vi "Module Execution Main.vi"(8 "error in":errorcluster, 10 "response queue":T1, 11 "command queue":T1) -> (0 "error out":errorcluster)   [LabVIEW 2013, in "module execution process.lvlib"]
doc: "This process allows a user to initialize, start, stop, monitor, and repeat using a message queue without stopping the main application. This process can be useful when you want to support the control of this target by one or more connected hosts."
uses:
  module execution process.lvlib
  <vilib>/NI/AMC/Message Queue.ctl
  <vilib>/NI/AMC/Message.ctl
  <vilib>/NI/Tools/Keyed Array/KeyedArray.ctl
  <vilib>/NI/Module Execution Interface/Engine Runtime/Engine Runtime Interface.lvclass
  <vilib>/NI/Configuration Framework/class discovery singleton/class discovery singleton methods.ctl
  SubVIs/configuration elements.ctl
  <vilib>/NI/Tag Bus Data Framework/Framework Configuration Classes/platypus configuration/engines cluster.ctl
  <vilib>/NI/Module Execution Interface/Engine Configuration/engine configuration.lvclass
  <vilib>/NI/Tag Bus Module Framework/module configuration/TBM module configuration.lvclass
  <vilib>/NI/Tag Bus Module Framework/runtime/TBM module execution interface.lvclass
  SubVIs/engine status data.ctl
  <vilib>/NI/Module Execution Interface/Engine Runtime/Execution States.ctl
  <vilib>/NI/AMC/Read Termination Message.vi
  <vilib>/NI/AMC/Create Single Message.vi
  <vilib>/NI/AMC/Globals.vi
  <vilib>/NI/Configuration Framework/class discovery singleton/class discovery singleton.lvlib
  <vilib>/NI/AMC/AMC.lvlib
  <vilib>/NI/Tag Bus Module Framework/FPGA manager/methods.ctl
  <vilib>/NI/Tag Bus Module Framework/FPGA manager/FPGA manager.lvlib
  <vilib>/userdefined/High Color/nirio_resource_hc.ctl
  <vilib>/rvi/interface/nirviOpenFPGA/nirviOpenFPGA.xnode
  <vilib>/NI/Tag Bus Data Framework/Framework Configuration Classes/target runtime/PL_Target Runtime.lvclass
  <vilib>/NI/Tag Bus Data Framework/Framework Configuration Classes/platypus configuration/PLConfigurationSerializer.lvlib
  <vilib>/NI/Configuration Framework/tree serializer/NISE_CEF_TreeSerializer.lvlib
  <vilib>/NI/Tag Bus Data Framework/Framework Configuration Classes/flattened data interface/PL_Serialization Interface.lvlib
  <vilib>/NI/Tools/Keyed Array/Tools_KeyedArray.lvlib
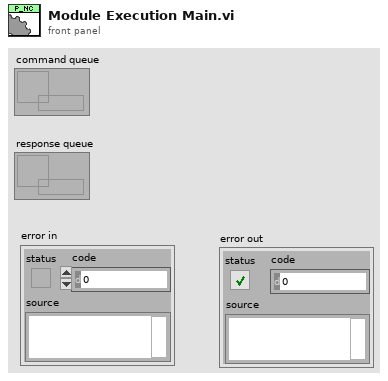
[diagram p1: front panel]
types:
  T1 = typedef "AMC.lvlib/Message Queue.ctl" = refnum<queue>
  T2 = typedef "class discovery singleton.lvlib/class discovery singleton methods.ctl" = enum16{"add search paths", "load class by name", "list available classes", "get class path"}
  T3 = typedef "module execution process.lvlib/configuration elements.ctl" = cluster{"Name":string, "opened?":bool, "configuration":T4, "engine":refnum<class "Engine Runtime Interface.lvclass">, "modules":refnum<class "TBM module execution interface.lvclass">[]}
  T4 = typedef "PLConfigurationSerializer.lvlib/engines cluster.ctl" = cluster{"engine configuration":refnum<class "engine configuration.lvclass">, "modules":refnum<class "TBM module configuration.lvclass">[]}
  T5 = typedef "nirio_resource_hc.ctl" = tag
  T6 = typedef "FPGA manager.lvlib/methods.ctl" = enum16{"initialize bitfile", "cache bitfile", "locate bitfile", "close bitfile"}
  T7 = typedef "module execution process.lvlib/engine status data.ctl" = cluster{"Name":string, "Engine State":T8, "Engine Error":errorcluster}
  T8 = typedef "Engine Runtime Interface.lvclass/Execution States.ctl" = enum16{"Initializing", "Paused (Initialized)", "Running", "Set Safe Outputs", "Uninitializing", "Stopped (Uninitialized)", "Error (Uninitialized)", "Safe State (Uninitialized)", "Closed"}
  T9 = typedef "module execution process.lvlib/command commands to rtexe process.ctl" = enum16{"Initialize", "Load from File", "Load from String", "Open All Engines", "Open Single Engine", "Initialize All Engines", "Initialize Single Engine", "Start All", "Start Single", "Pause All", "Pause Single", "Stop All", "Stop Single", "Close All", "Close Single", "Set Safe State All", "Set Safe State Single", "Get Status", "Exit", "Error", "Load Bitfile", "Unload Bitfile", "Add Search Paths"}
  T10 = typedef "NISE_CEF_TreeSerializer.lvlib/base file format.ctl" = cluster{"version":string, "data":string}
  T11 = typedef "NISE_CEF_TreeSerializer.lvlib/flat hierarchy.ctl" = cluster{"hierarchy structure":T12, "instance data":T14[]}
  T12 = typedef "NISE_CEF_TreeSerializer.lvlib/full hierarchy.ctl" = cluster{"root":string, "hierarchy":T13[]}
  T13 = typedef "NISE_CEF_TreeSerializer.lvlib/hierarchy element.ctl" = cluster{"current node":string, "children":string[]}
  T14 = typedef "NISE_CEF_TreeSerializer.lvlib/instance data.ctl" = cluster{"ID":string, "Alias":string, "class":string, "version":string, "data":string}
  T15 = typedef "PLConfigurationSerializer.lvlib/targets cluster.ctl" = cluster{"Target Configuration":refnum<class "PL_Target Configuration.lvclass">, "engines":T4[]}
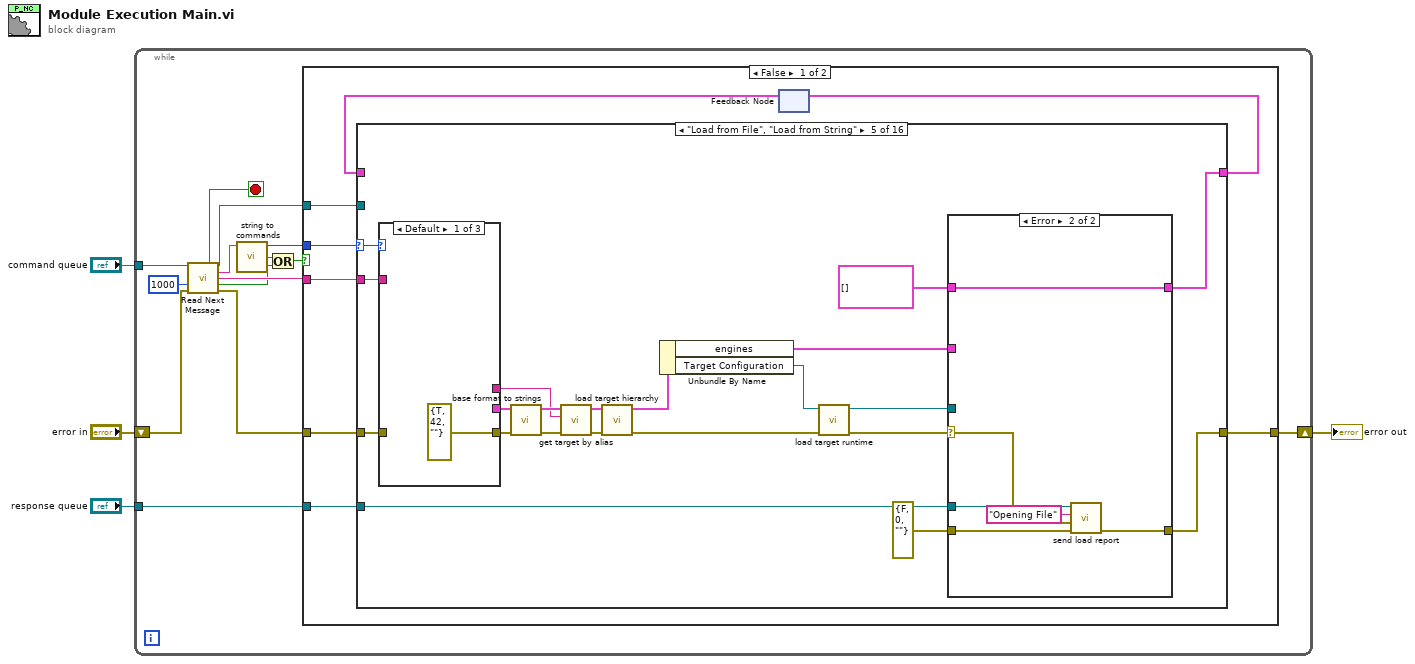
[diagram p0: block diagram]
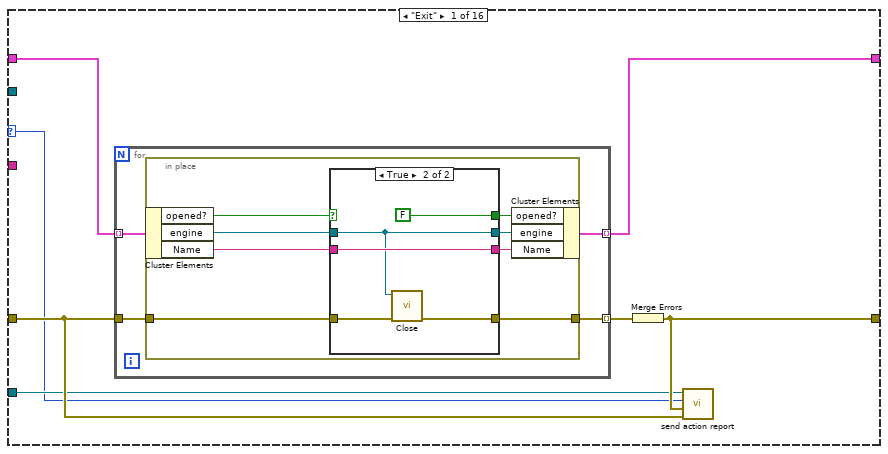
[diagram p2: hidden frame]
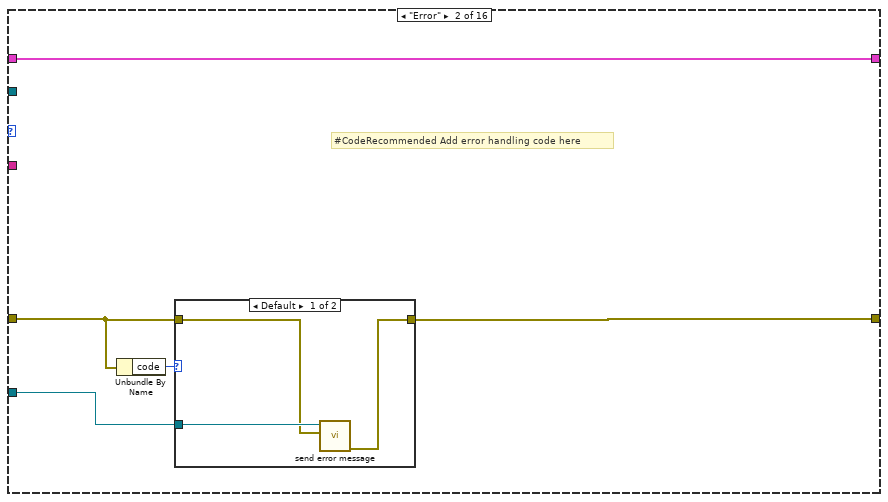
[diagram p4: hidden frame]
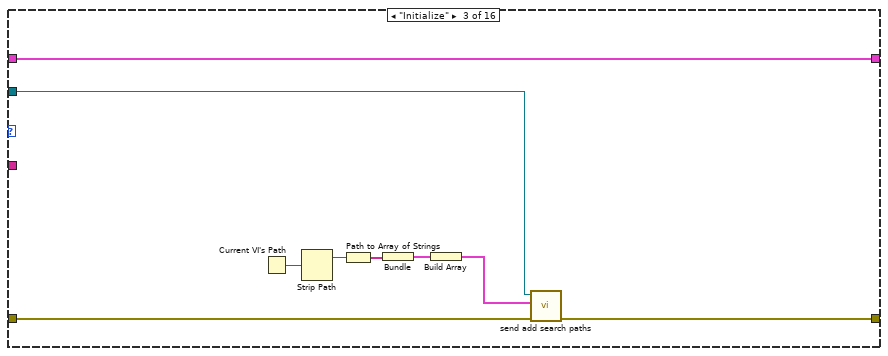
[diagram p6: hidden frame]
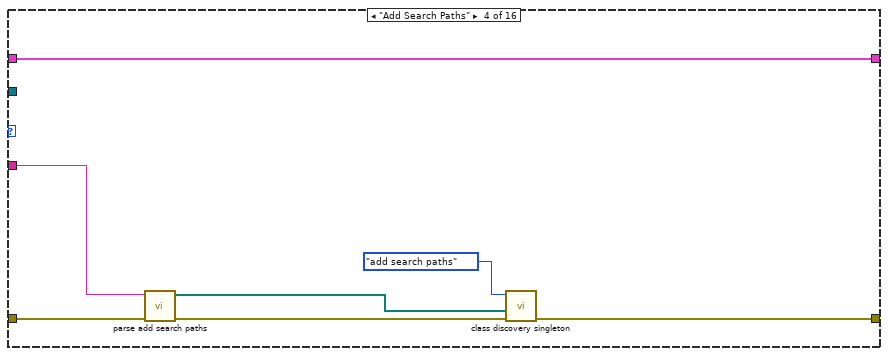
[diagram p7: hidden frame]
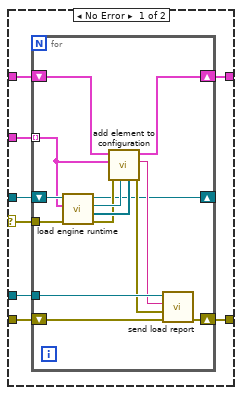
[diagram p8: hidden frame]
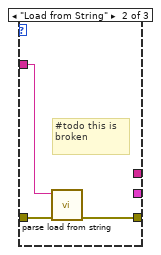
[diagram p9: hidden frame]
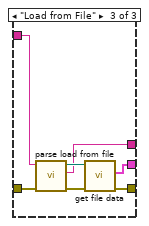
[diagram p10: hidden frame]
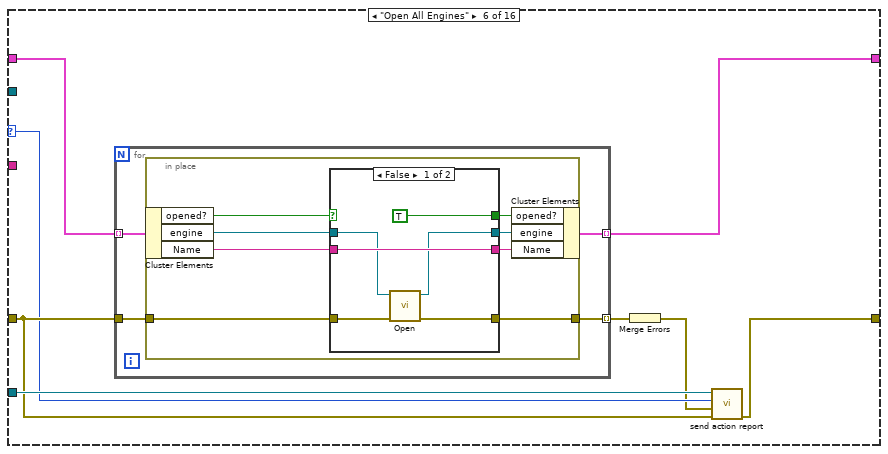
[diagram p11: hidden frame]
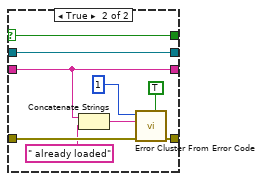
[diagram p12: hidden frame]
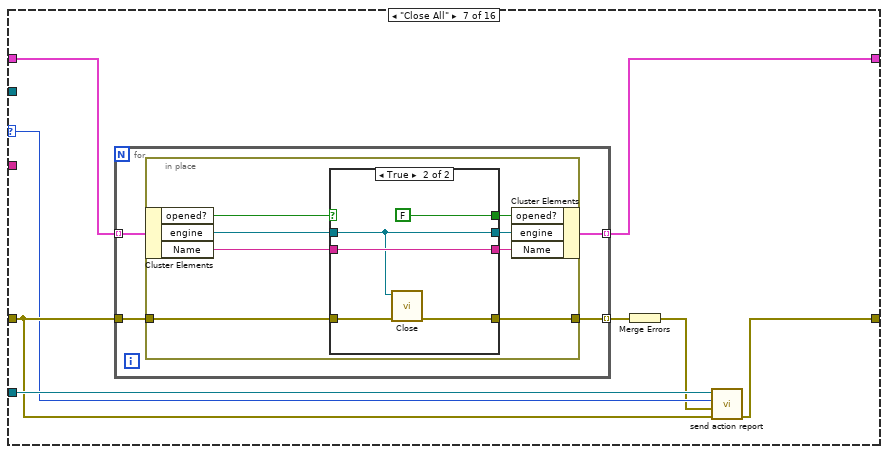
[diagram p13: hidden frame]
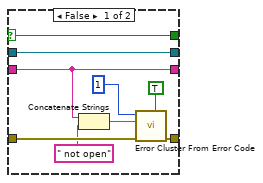
[diagram p14: hidden frame]
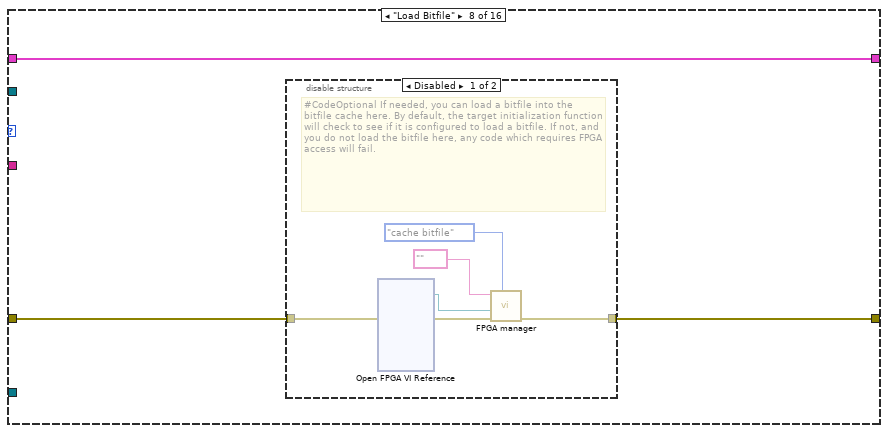
[diagram p15: hidden frame]
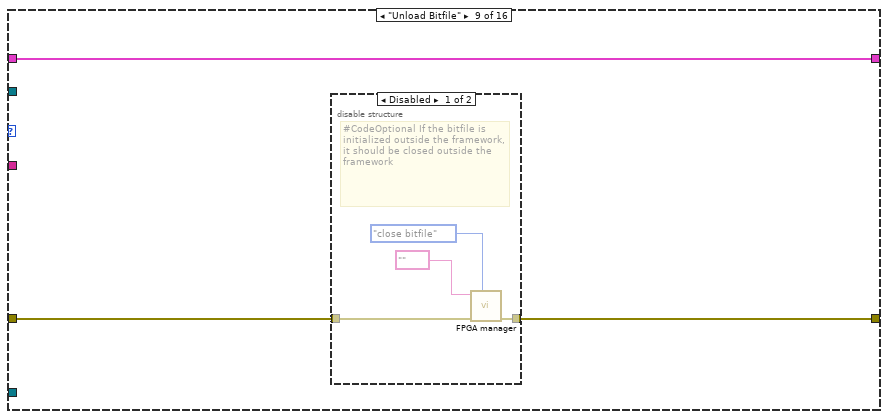
[diagram p17: hidden frame]
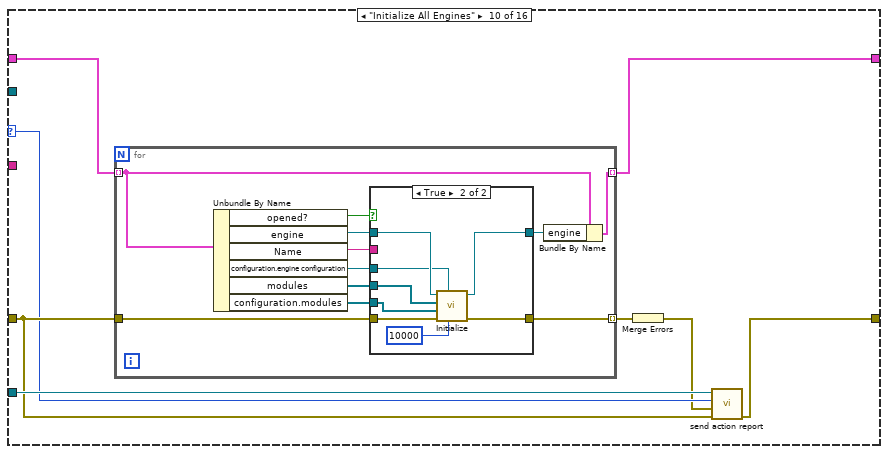
[diagram p19: hidden frame]
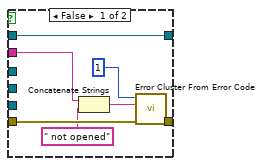
[diagram p20: hidden frame]
diagram:
  n1 = while {
    tunnel: "command queue" -> [w16]
    shift-right: [w18] -> w1
    shift-left: "error in" -> [w13]
    tunnel: "response queue" -> [w17]
    stop <- w15 stop-if-true
    n2 = call <vilib>:"Read Next Message.vi"("message queue in"=w16, "timeout (1 ms)"=1000, "error in"=w13) -> ("exit process?"=w15:bool, "message queue out"=w5:T1, "message name"=w10:string, "message value"=w14:string, "timed out?"=w8:bool, "error out"=w12:errorcluster)  [unwired: 5 in, 2 out]
    n3 = call "string to commands.vi"("command string"=w10) -> ("invalid"=w9:bool, "commands"=w6:T9)  [unwired: 9 in]
    n4 = Or(x=w9, y=w8) -> (x .or. y?=w7:bool)
    n5 = case shown="False" w7 {
      tunnel: w14 -> [w26 _]
      tunnel: [w25 w575] -> w18
      tunnel: w17 -> [w24 _]
      tunnel: w12 -> [w23 w575]
      tunnel: w6 -> [w22 _]
      tunnel: w5 -> [w21 _]
      frame False {
        n6 = feedback #1() -> (w19:T3[])  [unwired: 1 in]
        n7 = case shown="\"Load from File\", \"Load from String\"" w22 {
          selector: w22 -> [w27 _ _ _ w97 w140 w175 _ _ w227 w260 w319 w377 w434 w479 _]
          tunnel: w26 -> [_ _ _ w72 w99 _ _ _ _ _ _ w316 w374 w431 w486 _]
          tunnel: [w32 w59 w71 w78 w96 w145 w180 w210 w220 w232 w266 w322 w380 w437 w491 w551] -> w20
          tunnel: w19 -> [w33 w59 w71 w78 _ w146 w181 w210 w220 w233 w267 w323 w381 w438 w492 w552]
          tunnel: [w30 w56 w69 w76 w95 w142 w177 w208 w218 w229 w263 w320 w378 w435 w489 w549] -> w25
          tunnel: w23 -> [w29 w57 w70 w75 w98 w143 w178 w209 w219 w230 w264 w318 w376 w433 w488 w550]
          tunnel: w24 -> [w28 w55 _ _ w94 w144 w179 _ _ w231 w265 w321 w379 w436 w490 w548]
          tunnel: w21 -> [_ _ w68 _ _ _ _ _ _ _ _ _ _ _ _ _]
          frame "Exit" {
            n8 = for {
              tunnel: w33 -> [w37] mode=indexing
              tunnel: [w36] -> w32 mode=indexing
              tunnel: w29 -> [w35]
              tunnel: [w34] -> w31 mode=indexing
              n9 = in-place {
                in-place-border: w35 -> [w42]
                in-place-border: [w41] -> w34
                n10 = in-place-cluster #2(w37) -> ("opened?"=w45:bool, "engine"=w44:refnum<class "Engine Runtime Interface.lvclass">, "Name"=w40:string)
                n11 = case shown="True" w45 {
                  selector: w45 -> [w46 _]
                  tunnel: w44 -> [w49 w50]
                  tunnel: [w49 w50] -> w43
                  tunnel: w42 -> [w48 w52]
                  tunnel: [w48 w51] -> w41
                  tunnel: w40 -> [w47 w54]
                  tunnel: [w47 w54] -> w39
                  tunnel: [w46 FALSE ("opened?")] -> w38
                  frame False {
                  }
                  frame True {
                    n12 = call-dynamic "Close.vi"("error in"=w52, "Engine Runtime Interface in"=w50) -> ("error out"=w51:errorcluster)  [unwired: 9 in]
                  }
                }
                n13 = in-place-cluster #2("opened?"=w38, "engine"=w43, "Name"=w39) -> (w36:T3)
              }
            }
            n14 = Merge Errors(w31) -> (w30:errorcluster)
            n15 = call "send action report.vi"("error in"=w29, "command error"=w30, "commands"=w27, "message queue in"=w28) -> ()  [unwired: 6 in, 2 out]
          }
          frame "Error" {
            # "#CodeRecommended Add error handling code here"
            n16 = Unbundle By Name(w57) -> ("code"=w58:i32)
            n17 = case shown="Default" w58 {
              tunnel: w57 -> [w60 _]
              tunnel: [w61 _] -> w56
              tunnel: w55 -> [w62 _]
              frame Default {
                n18 = call "send error message.vi"("error to send"=w60, "message queue in"=w62) -> ("error out"=w61:errorcluster)  [unwired: 8 in, 1 out]
              }
              frame 538255 {
                # "Ignore this timeout error for now."
              }
            }
          }
          frame "Initialize" {
            n19 = Current VI's Path() -> (path=w67:path)
            n20 = Strip Path(path=w67) -> (stripped path=w66:path)  [unwired: 1 out]
            n21 = Path to Array of Strings(0:w66) -> (2:w65:string[])  [unwired: 1 out]
            n22 = Bundle("array of strings"=w65) -> (w64:cluster{"array of strings":string[]})  [unwired: 1 in]
            n23 = Build Array(w64) -> (w63:cluster{"array of strings":string[]}[])
            n24 = call "send add search paths.vi"("error in"=w70, "search paths"=w63, "message queue in"=w68) -> ("error out"=w69:errorcluster)  [unwired: 7 in, 1 out]
          }
          frame "Add Search Paths" {
            n25 = call "parse add search paths.vi"("error in"=w75, "message data"=w72) -> ("error out"=w74:errorcluster, "paths"=w73:path[])  [unwired: 8 in]
            n26 = call <vilib>:"class discovery singleton.vi"("error in"=w74, "Plugin Search Paths"=w73, "method"=class_discovery_singleton_methods."add search paths") -> ("error out"=w76:errorcluster)  [unwired: 5 in, 3 out]
          }
          frame "Load from File", "Load from String" {
            n27 = case shown="Default" w97 {
              tunnel: w99 -> [_ w129 w137]
              tunnel: w98 -> [_ w131 w138]
              tunnel: [errorcluster {"status"=TRUE, "code"=42, "source"=""} ("error out") w130 w134] -> w86
              tunnel: [_ _ w132] -> w79
              tunnel: [_ _ w133] -> w87
              frame Default {
              }
              frame "Load from String" {
                # "#todo this is broken"
                n28 = call "parse load from string.vi"("error in"=w131, "message data"=w129) -> ("error out"=w130:errorcluster)  [unwired: 7 in, 2 out]
              }
              frame "Load from File" {
                n29 = call "parse load from file.vi"("error in"=w138, "message data"=w137) -> ("error out"=w135:errorcluster, "target alias"=w132:string, "path"=w136:path)  [unwired: 7 in]
                n30 = call <vilib>:"get file data.vi"("error in"=w135, "Path"=w136) -> ("error out"=w134:errorcluster, "format"=w133:T10)  [unwired: 8 in]
              }
            }
            n31 = call <vilib>:"base format to strings.vi"("error in"=w86, "format"=w87) -> ("error out"=w81:errorcluster, "data"=w83:T11)  [unwired: 8 in]
            n32 = call <vilib>:"get target by alias.vi"("error in"=w81, "alias"=w79, "system hierarchy"=w83) -> ("error out"=w80:errorcluster, "target hierarchy"=w82:T11)  [unwired: 7 in]
            n33 = call <vilib>:"load target hierarchy.vi"("error in"=w80, "target hierarchy"=w82) -> ("error out"=w84:errorcluster, "targets cluster out"=w85:T15)  [unwired: 8 in]
            n34 = Unbundle By Name(w85) -> ("engines"=w92:T4[], "Target Configuration"=w93:refnum<class "PL_Target Configuration.lvclass">)
            n35 = call <vilib>:"load target runtime.vi"("error in"=w84, "target configuration"=w93) -> ("error out"=w88:errorcluster, "target runtime"=w91:refnum<class "PL_Target Runtime.lvclass">)  [unwired: 8 in]
            n36 = case shown="Error" w88 {
              selector: w88 -> [w100 w126]
              tunnel: [w107 w127] -> w96
              tunnel: [w106 w124] -> w95
              tunnel: w94 -> [w105 w123]
              tunnel: w92 -> [w104 _]
              tunnel: w91 -> [w103 _]
              tunnel: errorcluster {"status"=FALSE, "code"=0, "source"=""} ("error out") -> [w102 w125]
              tunnel: T3[] [] ("Configuration out") -> [w101 w127]
              frame No Error {
                n37 = for {
                  shift-right: [w121] -> w107
                  shift-left: w101 -> [w120]
                  shift-right: [w118] -> w106
                  shift-left: w102 -> [w115]
                  tunnel: w105 -> [w119]
                  tunnel: w104 -> [w108] mode=indexing
                  shift-right: [w109] -> _
                  shift-left: w103 -> [w114]
                  tunnel: w100 -> [w113]
                  n38 = call <vilib>:"load engine runtime.vi"("error in"=w113, "engine configuration in"=w108, "Target Runtime in"=w114) -> ("error out"=w110:errorcluster, "Module Runtime Objects"=w111:refnum<class "TBM module execution interface.lvclass">[], "Engine Runtime Object"=w112:refnum<class "Engine Runtime Interface.lvclass">, "Target Runtime out"=w109:refnum<class "PL_Target Runtime.lvclass">)  [unwired: 5 in]
                  n39 = call "add element to configuration.vi"("Module Runtime Objects"=w111, "Engine Runtime Object"=w112, "error in"=w110, "engine configuration in"=w108, "Configuration in"=w120) -> ("error out"=w116:errorcluster, "engine loaded"=w117:string, "Configuration out"=w121:T3[])  [unwired: 4 in]
                  n40 = call "send load report.vi"("error in"=w115, "load error"=w116, "engine loaded"=w117, "message queue in"=w119) -> ("error out"=w118:errorcluster)  [unwired: 6 in, 1 out]
                }
              }
              frame Error {
                n41 = call "send load report.vi"("error in"=w125, "load error"=w126, "engine loaded"="Opening File", "message queue in"=w123) -> ("error out"=w124:errorcluster)  [unwired: 6 in, 1 out]
              }
            }
          }
          frame "Open All Engines" {
            n42 = for {
              tunnel: w146 -> [w150] mode=indexing
              tunnel: [w149] -> w145 mode=indexing
              tunnel: w143 -> [w148]
              tunnel: [w147] -> w141 mode=indexing
              n43 = in-place {
                in-place-border: w148 -> [w155]
                in-place-border: [w154] -> w147
                n44 = in-place-cluster #3(w150) -> ("opened?"=w158:bool, "engine"=w157:refnum<class "Engine Runtime Interface.lvclass">, "Name"=w153:string)
                n45 = case shown="False" w158 {
                  selector: w158 -> [_ w165]
                  tunnel: w157 -> [w161 w173]
                  tunnel: [w160 w173] -> w156
                  tunnel: w155 -> [w164 w172]
                  tunnel: [w163 w171] -> w154
                  tunnel: w153 -> [w162 w166]
                  tunnel: [w162 w166] -> w152
                  tunnel: [TRUE ("opened?") w165] -> w151
                  frame False {
                    n46 = call-dynamic "Open.vi"("error in"=w164, "Engine Runtime Interface in"=w161) -> ("error out"=w163:errorcluster, "Engine Runtime Interface out"=w160:refnum<class "Engine Runtime Interface.lvclass">)  [unwired: 8 in]
                  }
                  frame True {
                    n47 = Concatenate Strings(w166, " already loaded" ("string")) -> (w168:string)
                    n48 = call <vilib>:"Error Cluster From Error Code.vi"("is warning? (False)"=TRUE, "error in (no error)"=w172, "error message (\"\")"=w168, "error code (0)"=1) -> ("error out"=w171:errorcluster)  [unwired: 5 in]
                  }
                }
                n49 = in-place-cluster #3("opened?"=w151, "engine"=w156, "Name"=w152) -> (w149:T3)
              }
            }
            n50 = Merge Errors(w141) -> (w139:errorcluster)
            n51 = call "send action report.vi"("error in"=w143, "command error"=w139, "commands"=w140, "message queue in"=w144) -> ("error out"=w142:errorcluster)  [unwired: 6 in, 1 out]
          }
          frame "Close All" {
            n52 = for {
              tunnel: w181 -> [w185] mode=indexing
              tunnel: [w184] -> w180 mode=indexing
              tunnel: w178 -> [w183]
              tunnel: [w182] -> w176 mode=indexing
              n53 = in-place {
                in-place-border: w183 -> [w190]
                in-place-border: [w189] -> w182
                n54 = in-place-cluster #4(w185) -> ("opened?"=w193:bool, "engine"=w192:refnum<class "Engine Runtime Interface.lvclass">, "Name"=w188:string)
                n55 = case shown="True" w193 {
                  selector: w193 -> [w194 _]
                  tunnel: w192 -> [w202 w203]
                  tunnel: [w202 w203] -> w191
                  tunnel: w190 -> [w201 w205]
                  tunnel: [w200 w204] -> w189
                  tunnel: w188 -> [w195 w207]
                  tunnel: [w195 w207] -> w187
                  tunnel: [w194 FALSE ("opened?")] -> w186
                  frame False {
                    n56 = Concatenate Strings(w195, " not open" ("string")) -> (w197:string)
                    n57 = call <vilib>:"Error Cluster From Error Code.vi"("is warning? (False)"=TRUE, "error in (no error)"=w201, "error message (\"\")"=w197, "error code (0)"=1) -> ("error out"=w200:errorcluster)  [unwired: 5 in]
                  }
                  frame True {
                    n58 = call-dynamic "Close.vi"("error in"=w205, "Engine Runtime Interface in"=w203) -> ("error out"=w204:errorcluster)  [unwired: 9 in]
                  }
                }
                n59 = in-place-cluster #4("opened?"=w186, "engine"=w191, "Name"=w187) -> (w184:T3)
              }
            }
            n60 = Merge Errors(w176) -> (w174:errorcluster)
            n61 = call "send action report.vi"("error in"=w178, "command error"=w174, "commands"=w175, "message queue in"=w179) -> ("error out"=w177:errorcluster)  [unwired: 6 in, 1 out]
          }
          frame "Load Bitfile" {
            n62 = disable-structure shown="Disabled" {
              disable-tunnel: [w212 w217] -> w208
              disable-tunnel: w209 -> [w211 w217]
              frame Disabled {
                # "#CodeOptional If needed, you can load a bitfile into the bitfile cache here. By default, the target initialization function will check to see if it is configured to load a bitfile. If not, and you do not load the bitfile here, any code which requires FPGA access will fail."
                n63 = xnode "Open FPGA VI Reference"("error in"=w211) -> ("FPGA VI Reference Out"=w215:refnum<k20>, "error out"=w216:errorcluster)  [unwired: 1 in]
                n64 = call <vilib>:"FPGA manager.vi"("action"=methods."cache bitfile", "error in"=w216, "bitfile to cache"=w215, "RIO resource"=T5 "") -> ("error out"=w212:errorcluster)  [unwired: 5 in, 2 out]
              }
              frame Enabled {
              }
            }
          }
          frame "Unload Bitfile" {
            n65 = disable-structure shown="Disabled" {
              disable-tunnel: w219 -> [w222 w225]
              disable-tunnel: [w221 w225] -> w218
              frame Disabled {
                # "#CodeOptional If the bitfile is initialized outside the framework, it should be closed outside the framework"
                n66 = call <vilib>:"FPGA manager.vi"("action"=methods."close bitfile", "error in"=w222, "RIO resource"=T5 "") -> ("error out"=w221:errorcluster)  [unwired: 6 in, 2 out]
              }
              frame Enabled {
              }
            }
          }
          frame "Initialize All Engines" {
            n67 = for {
              tunnel: w233 -> [w244] mode=indexing
              tunnel: [w243] -> w232 mode=indexing
              tunnel: w230 -> [w242]
              tunnel: [w241] -> w228 mode=indexing
              n68 = Unbundle By Name(w244) -> ("opened?"=w240:bool, "engine"=w239:refnum<class "Engine Runtime Interface.lvclass">, "Name"=w237:string, "configuration.engine configuration"=w236:refnum<class "engine configuration.lvclass">, "modules"=w235:refnum<class "TBM module execution interface.lvclass">[], "configuration.modules"=w234:refnum<class "TBM module configuration.lvclass">[])
              n69 = case shown="True" w240 {
                tunnel: w239 -> [w251 w256]
                tunnel: [w251 w257] -> w238
                tunnel: w242 -> [w250 w258]
                tunnel: [w249 w259] -> w241
                tunnel: w237 -> [w245 _]
                tunnel: w236 -> [_ w255]
                tunnel: w235 -> [_ w254]
                tunnel: w234 -> [_ w253]
                frame False {
                  n70 = Concatenate Strings(w245, " not opened" ("string")) -> (w247:string)
                  n71 = call <vilib>:"Error Cluster From Error Code.vi"("error in (no error)"=w250, "error message (\"\")"=w247, "error code (0)"=1) -> ("error out"=w249:errorcluster)  [unwired: 6 in]
                }
                frame True {
                  n72 = call-dynamic "Initialize.vi"("timeout in ms"=10000, "Engine Configuration"=w255, "error in"=w258, "module Configurations"=w253, "modules"=w254, "Engine Runtime Interface in"=w256) -> ("error out"=w259:errorcluster, "Engine Runtime Interface out"=w257:refnum<class "Engine Runtime Interface.lvclass">)  [unwired: 4 in]
                }
              }
              n73 = Bundle By Name(cluster=w244, "engine"=w238) -> (w243:T3)
            }
            n74 = Merge Errors(w228) -> (w226:errorcluster)
            n75 = call "send action report.vi"("error in"=w230, "command error"=w226, "commands"=w227, "message queue in"=w231) -> ("error out"=w229:errorcluster)  [unwired: 6 in, 1 out]
          }
          frame "Start All", "Pause All", "Stop All", "Set Safe State All" {
            n76 = for {
              tunnel: w267 -> [w276] mode=indexing
              tunnel: [w275] -> w266 mode=indexing
              tunnel: w264 -> [w274]
              tunnel: [w273] -> w262 mode=indexing
              tunnel: w260 -> [w268]
              n77 = Unbundle By Name(w276) -> ("opened?"=w272:bool, "engine"=w271:refnum<class "Engine Runtime Interface.lvclass">, "Name"=w269:string)
              n78 = case shown="True" w272 {
                tunnel: w271 -> [w283 w285]
                tunnel: [w283 w286] -> w270
                tunnel: w274 -> [w282 w288]
                tunnel: [w281 w287] -> w273
                tunnel: w269 -> [w277 _]
                tunnel: w268 -> [_ w284]
                frame False {
                  n79 = Concatenate Strings(w277, " not opened" ("string")) -> (w279:string)
                  n80 = call <vilib>:"Error Cluster From Error Code.vi"("error in (no error)"=w282, "error message (\"\")"=w279, "error code (0)"=1) -> ("error out"=w281:errorcluster)  [unwired: 6 in]
                }
                frame True {
                  n81 = case shown="\"Start All\"" w284 {
                    tunnel: w288 -> [w291 w297 w301 w305 w309]
                    tunnel: [w292 w296 w300 w304 w308] -> w287
                    tunnel: [w293 w295 w299 w302 w307] -> w286
                    tunnel: w285 -> [w293 w294 w298 w303 w306]
                    frame Default {
                      n82 = call <vilib>:"Error Cluster From Error Code.vi"("error in (no error)"=w291, "error message (\"\")"="dev" ("error message (\"\")"), "error code (0)"=42) -> ("error out"=w292:errorcluster)  [unwired: 6 in]
                    }
                    frame "Start All" {
                      n83 = call-dynamic "Start.vi"("error in"=w297, "Engine Runtime Interface in"=w294) -> ("error out"=w296:errorcluster, "Engine Runtime Interface out"=w295:refnum<class "Engine Runtime Interface.lvclass">)  [unwired: 8 in]
                    }
                    frame "Pause All" {
                      n84 = call-dynamic "Pause.vi"("error in"=w301, "Engine Runtime Interface in"=w298) -> ("error out"=w300:errorcluster, "Engine Runtime Interface out"=w299:refnum<class "Engine Runtime Interface.lvclass">)  [unwired: 8 in]
                    }
                    frame "Stop All" {
                      n85 = call-dynamic "Stop.vi"("error in"=w305, "Engine Runtime Interface in"=w303) -> ("error out"=w304:errorcluster, "Engine Runtime Interface out"=w302:refnum<class "Engine Runtime Interface.lvclass">)  [unwired: 8 in]
                    }
                    frame "Set Safe State All" {
                      n86 = call-dynamic "Set Safe State.vi"("error in"=w309, "Engine Runtime Interface in"=w306) -> ("error out"=w308:errorcluster, "Engine Runtime Interface out"=w307:refnum<class "Engine Runtime Interface.lvclass">)  [unwired: 8 in]
                    }
                  }
                }
              }
              n87 = Bundle By Name(cluster=w276, "engine"=w270) -> (w275:T3)
            }
            n88 = Merge Errors(w262) -> (w261:errorcluster)
            n89 = call "send action report.vi"("error in"=w264, "command error"=w261, "commands"=w260, "message queue in"=w265) -> ("error out"=w263:errorcluster)  [unwired: 6 in, 1 out]
          }
          frame "Open Single Engine" {
            n90 = call "parse single action command.vi"("error in"=w318, "message data"=w316) -> ("error out"=w317:errorcluster, "engine name"=w315:string)  [unwired: 8 in]
            n91 = for {
              tunnel: w323 -> [w330] mode=indexing
              tunnel: [w329] -> w322 mode=indexing
              tunnel: w315 -> [w326]
              tunnel: [w325] -> w314 mode=indexing
              tunnel: w317 -> [w328]
              tunnel: [w327] -> w312
              stop <- w324 stop-if-true
              n92 = in-place {
                in-place-border: w328 -> [w337]
                in-place-border: [w336] -> w327
                in-place-border: w326 -> [w333]
                in-place-border: [w331] -> w325
                in-place-border: [w331] -> w324
                n93 = in-place-cluster #5(w330) -> ("opened?"=w340:bool, "engine"=w339:refnum<class "Engine Runtime Interface.lvclass">, "Name"=w332:string)
                n94 = Equal?(x=w332, y=w333) -> (x = y?=w331:bool)
                n95 = case shown="True" w331 {
                  tunnel: w340 -> [w344 w352]
                  tunnel: w339 -> [w343 w351]
                  tunnel: [w343 w350] -> w338
                  tunnel: w337 -> [w341 w349]
                  tunnel: [w341 w348] -> w336
                  tunnel: [w342 w347] -> w335
                  tunnel: [w344 w346] -> w334
                  tunnel: w332 -> [w342 w345]
                  frame False {
                  }
                  frame True {
                    n96 = case shown="False" w352 {
                      selector: w352 -> [_ w359]
                      tunnel: w351 -> [w355 w367]
                      tunnel: [w354 w367] -> w350
                      tunnel: w349 -> [w358 w366]
                      tunnel: [w357 w365] -> w348
                      tunnel: w345 -> [w356 w360]
                      tunnel: [w356 w360] -> w347
                      tunnel: [TRUE ("opened?") w359] -> w346
                      frame False {
                        n97 = call-dynamic "Open.vi"("error in"=w358, "Engine Runtime Interface in"=w355) -> ("error out"=w357:errorcluster, "Engine Runtime Interface out"=w354:refnum<class "Engine Runtime Interface.lvclass">)  [unwired: 8 in]
                      }
                      frame True {
                        n98 = Concatenate Strings(w360, " already loaded" ("string")) -> (w362:string)
                        n99 = call <vilib>:"Error Cluster From Error Code.vi"("is warning? (False)"=TRUE, "error in (no error)"=w366, "error message (\"\")"=w362, "error code (0)"=1) -> ("error out"=w365:errorcluster)  [unwired: 5 in]
                      }
                    }
                  }
                }
                n100 = in-place-cluster #5("opened?"=w334, "engine"=w338, "Name"=w335) -> (w329:T3)
              }
            }
            n101 = Or Array Elements(Boolean array=w314) -> (logical OR=w313:bool)
            n102 = Select(t=w312, s=w313, f=errorcluster {"status"=TRUE, "code"=1, "source"="Not found"}) -> (s? t:f=w311:errorcluster)
            n103 = call "send action report.vi"("error in"=w317, "command error"=w311, "commands"=w319, "message queue in"=w321) -> ("error out"=w320:errorcluster)  [unwired: 6 in, 1 out]
          }
          frame "Close Single" {
            n104 = call "parse single action command.vi"("error in"=w376, "message data"=w374) -> ("error out"=w375:errorcluster, "engine name"=w373:string)  [unwired: 8 in]
            n105 = for {
              tunnel: w381 -> [w388] mode=indexing
              tunnel: [w387] -> w380 mode=indexing
              tunnel: w373 -> [w384]
              tunnel: [w383] -> w372 mode=indexing
              tunnel: w375 -> [w386]
              tunnel: [w385] -> w370
              stop <- w382 stop-if-true
              n106 = in-place {
                in-place-border: w386 -> [w395]
                in-place-border: [w394] -> w385
                in-place-border: w384 -> [w391]
                in-place-border: [w389] -> w383
                in-place-border: [w389] -> w382
                n107 = in-place-cluster #6(w388) -> ("opened?"=w398:bool, "engine"=w397:refnum<class "Engine Runtime Interface.lvclass">, "Name"=w390:string)
                n108 = Equal?(x=w390, y=w391) -> (x = y?=w389:bool)
                n109 = case shown="True" w389 {
                  tunnel: w398 -> [w402 w410]
                  tunnel: w397 -> [w401 w409]
                  tunnel: [w401 w408] -> w396
                  tunnel: w395 -> [w399 w407]
                  tunnel: [w399 w406] -> w394
                  tunnel: [w400 w405] -> w393
                  tunnel: [w402 w404] -> w392
                  tunnel: w390 -> [w400 w403]
                  frame False {
                  }
                  frame True {
                    n110 = case shown="True" w410 {
                      selector: w410 -> [w411 _]
                      tunnel: w409 -> [w419 w420]
                      tunnel: [w419 w420] -> w408
                      tunnel: w407 -> [w418 w421]
                      tunnel: [w417 w422] -> w406
                      tunnel: w403 -> [w412 w424]
                      tunnel: [w412 w424] -> w405
                      tunnel: [w411 FALSE ("opened?")] -> w404
                      frame False {
                        n111 = Concatenate Strings(w412, " not opened" ("string")) -> (w414:string)
                        n112 = call <vilib>:"Error Cluster From Error Code.vi"("is warning? (False)"=TRUE, "error in (no error)"=w418, "error message (\"\")"=w414, "error code (0)"=1) -> ("error out"=w417:errorcluster)  [unwired: 5 in]
                      }
                      frame True {
                        n113 = call-dynamic "Close.vi"("error in"=w421, "Engine Runtime Interface in"=w420) -> ("error out"=w422:errorcluster)  [unwired: 9 in]
                      }
                    }
                  }
                }
                n114 = in-place-cluster #6("opened?"=w392, "engine"=w396, "Name"=w393) -> (w387:T3)
              }
            }
            n115 = Or Array Elements(Boolean array=w372) -> (logical OR=w371:bool)
            n116 = Select(t=w370, s=w371, f=errorcluster {"status"=TRUE, "code"=1, "source"="Not found"}) -> (s? t:f=w369:errorcluster)
            n117 = call "send action report.vi"("error in"=w375, "command error"=w369, "commands"=w377, "message queue in"=w379) -> ("error out"=w378:errorcluster)  [unwired: 6 in, 1 out]
          }
          frame "Initialize Single Engine" {
            n118 = call "parse single action command.vi"("error in"=w433, "message data"=w431) -> ("error out"=w432:errorcluster, "engine name"=w430:string)  [unwired: 8 in]
            n119 = for {
              tunnel: w438 -> [w451] mode=indexing
              tunnel: [w450] -> w437 mode=indexing
              tunnel: w430 -> [w447]
              tunnel: [w446] -> w429 mode=indexing
              tunnel: w432 -> [w449]
              tunnel: [w448] -> w427
              stop <- w446 stop-if-true
              n120 = Unbundle By Name(w451) -> ("configuration.engine configuration"=w439:refnum<class "engine configuration.lvclass">, "opened?"=w445:bool, "engine"=w444:refnum<class "Engine Runtime Interface.lvclass">, "modules"=w440:refnum<class "TBM module execution interface.lvclass">[], "configuration.modules"=w441:refnum<class "TBM module configuration.lvclass">[], "Name"=w442:string)
              n121 = Equal?(x=w442, y=w447) -> (x = y?=w446:bool)
              n122 = case shown="True" w446 {
                tunnel: w445 -> [_ w462]
                tunnel: w444 -> [w453 w461]
                tunnel: [w453 w460] -> w443
                tunnel: w449 -> [w452 w459]
                tunnel: [w452 w458] -> w448
                tunnel: w442 -> [_ w457]
                tunnel: w441 -> [_ w456]
                tunnel: w440 -> [_ w455]
                tunnel: w439 -> [_ w454]
                frame False {
                }
                frame True {
                  n123 = case shown="True" w462 {
                    tunnel: w461 -> [w470 w476]
                    tunnel: [w470 w475] -> w460
                    tunnel: w459 -> [w469 w477]
                    tunnel: [w468 w474] -> w458
                    tunnel: w457 -> [w463 _]
                    tunnel: w456 -> [_ w473]
                    tunnel: w455 -> [_ w472]
                    tunnel: w454 -> [_ w471]
                    frame False {
                      n124 = Concatenate Strings(w463, " not opened" ("string")) -> (w465:string)
                      n125 = call <vilib>:"Error Cluster From Error Code.vi"("is warning? (False)"=TRUE, "error in (no error)"=w469, "error message (\"\")"=w465, "error code (0)"=1) -> ("error out"=w468:errorcluster)  [unwired: 5 in]
                    }
                    frame True {
                      n126 = call-dynamic "Initialize.vi"("timeout in ms"=10000, "Engine Configuration"=w471, "error in"=w477, "module Configurations"=w473, "modules"=w472, "Engine Runtime Interface in"=w476) -> ("error out"=w474:errorcluster, "Engine Runtime Interface out"=w475:refnum<class "Engine Runtime Interface.lvclass">)  [unwired: 4 in]
                    }
                  }
                }
              }
              n127 = Bundle By Name(cluster=w451, "engine"=w443) -> (w450:T3)
            }
            n128 = Or Array Elements(Boolean array=w429) -> (logical OR=w428:bool)
            n129 = Select(t=w427, s=w428, f=errorcluster {"status"=TRUE, "code"=1, "source"="Not found"}) -> (s? t:f=w426:errorcluster)
            n130 = call "send action report.vi"("error in"=w432, "command error"=w426, "commands"=w434, "message queue in"=w436) -> ("error out"=w435:errorcluster)  [unwired: 6 in, 1 out]
          }
          frame "Start Single", "Pause Single", "Stop Single", "Set Safe State Single" {
            n131 = call "parse single action command.vi"("error in"=w488, "message data"=w486) -> ("error out"=w487:errorcluster, "engine name"=w485:string)  [unwired: 8 in]
            n132 = for {
              tunnel: w492 -> [w503] mode=indexing
              tunnel: [w502] -> w491 mode=indexing
              tunnel: w485 -> [w499]
              tunnel: [w498] -> w484 mode=indexing
              tunnel: w487 -> [w501]
              tunnel: [w500] -> w482
              tunnel: w479 -> [w493]
              stop <- w498 stop-if-true
              n133 = Unbundle By Name(w503) -> ("opened?"=w497:bool, "engine"=w496:refnum<class "Engine Runtime Interface.lvclass">, "Name"=w494:string)
              n134 = Equal?(x=w494, y=w499) -> (x = y?=w498:bool)
              n135 = case shown="True" w498 {
                tunnel: w497 -> [_ w512]
                tunnel: w496 -> [w505 w511]
                tunnel: [w505 w510] -> w495
                tunnel: w501 -> [w504 w509]
                tunnel: [w504 w508] -> w500
                tunnel: w494 -> [_ w507]
                tunnel: w493 -> [_ w506]
                frame False {
                }
                frame True {
                  n136 = case shown="True" w512 {
                    tunnel: w511 -> [w520 w523]
                    tunnel: [w520 w524] -> w510
                    tunnel: w509 -> [w519 w522]
                    tunnel: [w518 w525] -> w508
                    tunnel: w507 -> [w513 _]
                    tunnel: w506 -> [_ w521]
                    frame False {
                      n137 = Concatenate Strings(w513, " not opened" ("string")) -> (w515:string)
                      n138 = call <vilib>:"Error Cluster From Error Code.vi"("is warning? (False)"=TRUE, "error in (no error)"=w519, "error message (\"\")"=w515, "error code (0)"=1) -> ("error out"=w518:errorcluster)  [unwired: 5 in]
                    }
                    frame True {
                      n139 = case shown="\"Set Safe State Single\"" w521 {
                        tunnel: w522 -> [w528 w534 w538 w542 w546]
                        tunnel: [w529 w533 w537 w541 w545] -> w525
                        tunnel: [w530 w532 w536 w540 w543] -> w524
                        tunnel: w523 -> [w530 w531 w535 w539 w544]
                        frame Default {
                          n140 = call <vilib>:"Error Cluster From Error Code.vi"("error in (no error)"=w528, "error message (\"\")"="dev" ("error message (\"\")"), "error code (0)"=42) -> ("error out"=w529:errorcluster)  [unwired: 6 in]
                        }
                        frame "Start Single" {
                          n141 = call-dynamic "Start.vi"("error in"=w534, "Engine Runtime Interface in"=w531) -> ("error out"=w533:errorcluster, "Engine Runtime Interface out"=w532:refnum<class "Engine Runtime Interface.lvclass">)  [unwired: 8 in]
                        }
                        frame "Pause Single" {
                          n142 = call-dynamic "Pause.vi"("error in"=w538, "Engine Runtime Interface in"=w535) -> ("error out"=w537:errorcluster, "Engine Runtime Interface out"=w536:refnum<class "Engine Runtime Interface.lvclass">)  [unwired: 8 in]
                        }
                        frame "Set Safe State Single" {
                          n143 = call-dynamic "Set Safe State.vi"("error in"=w542, "Engine Runtime Interface in"=w539) -> ("error out"=w541:errorcluster, "Engine Runtime Interface out"=w540:refnum<class "Engine Runtime Interface.lvclass">)  [unwired: 8 in]
                        }
                        frame "Stop Single" {
                          n144 = call-dynamic "Stop.vi"("error in"=w546, "Engine Runtime Interface in"=w544) -> ("error out"=w545:errorcluster, "Engine Runtime Interface out"=w543:refnum<class "Engine Runtime Interface.lvclass">)  [unwired: 8 in]
                        }
                      }
                    }
                  }
                }
              }
              n145 = Bundle By Name(cluster=w503, "engine"=w495) -> (w502:T3)
            }
            n146 = Or Array Elements(Boolean array=w484) -> (logical OR=w483:bool)
            n147 = Select(t=w482, s=w483, f=errorcluster {"status"=TRUE, "code"=1, "source"="Not found"}) -> (s? t:f=w481:errorcluster)
            n148 = call "send action report.vi"("error in"=w487, "command error"=w481, "commands"=w479, "message queue in"=w490) -> ("error out"=w489:errorcluster)  [unwired: 6 in, 1 out]
          }
          frame "Get Status" {
            n149 = for {
              tunnel: w552 -> [w563] mode=indexing
              tunnel: [w562] -> w551 mode=indexing
              tunnel: w550 -> [w561]
              tunnel: [w557] -> w547 mode=indexing
              n150 = Unbundle By Name(w563) -> ("Name"=w553:string, "opened?"=w560:bool, "engine"=w559:refnum<class "Engine Runtime Interface.lvclass">)
              n151 = case shown="True" w560 {
                tunnel: w559 -> [w565 w572]
                tunnel: [w565 w569] -> w558
                tunnel: w561 -> [_ w574]
                tunnel: [Execution_States."Closed" ("Engine State") w570] -> w554
                tunnel: [_ w567] -> w555
                frame False {
                }
                frame True {
                  n152 = call-dynamic "Get State.vi"("error in"=w574, "Engine Runtime Interface in"=w572) -> ("error out"=w573:errorcluster, "Engine State"=w570:T8, "Engine Runtime Interface out"=w571:refnum<class "Engine Runtime Interface.lvclass">)  [unwired: 7 in]
                  n153 = call-dynamic "Read Buffered Error.vi"("error in"=w573, "Engine Runtime Interface in"=w571) -> ("error out"=w566:errorcluster, "Engine Error"=w568:errorcluster, "Engine Runtime Interface out"=w569:refnum<class "Engine Runtime Interface.lvclass">)  [unwired: 7 in]
                  n154 = Merge Errors(w568, w566) -> (w567:errorcluster)
                }
              }
              n155 = Bundle By Name(cluster=w563, "engine"=w558) -> (w562:T3)
              n156 = Bundle(cluster=T7 {"Name"="", "Engine State"=enum."Initializing", "Engine Error"={"status"=FALSE, "code"=0, "source"=""}}, "Name"=w553, "Engine State"=w554, "Engine Error"=w555) -> (w557:T7)
            }
            n157 = call "send engine statuses.vi"("error in"=w550, "statuses"=w547, "message queue in"=w548) -> ("error out"=w549:errorcluster)  [unwired: 7 in, 1 out]
          }
        }
        n158 = feedback-in #1(w20) -> ()
      }
      frame True {
      }
    }
  }
  "error out" <- w1
